vi "GetRefExample.vi"() -> ()   [LabVIEW 2019]
uses:
  _get control reference by name.vi
  _get mutiple control reference by name.vi
panel:
  in  "error in":errorcluster
  out "error out":errorcluster
  in  "Important Tab Control":enum32{"Page 1", "Page 2"}(tab)
  in  "Not So Important Path":path
  in  "Important String":string
  in  "Important Sub Tab Control":enum32{"Page 1", "Page 2"}(tab)
  out "Important Chart":dbl(graph)
  in  "Important Table":string[][](table)
  in  "Important Path":path
  in  "Important Button":bool
  in  "Important Number":dbl
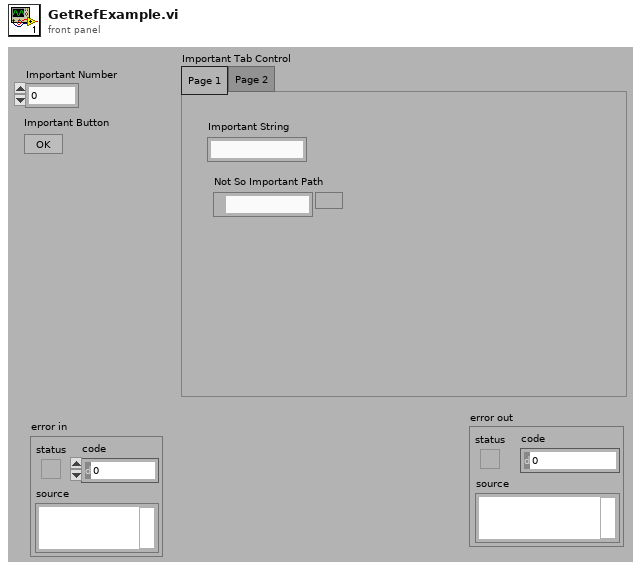
[diagram p1: front panel]
types:
  T1 = cluster{"ControlName":string, "ControlReference":refnum<vi>}[]
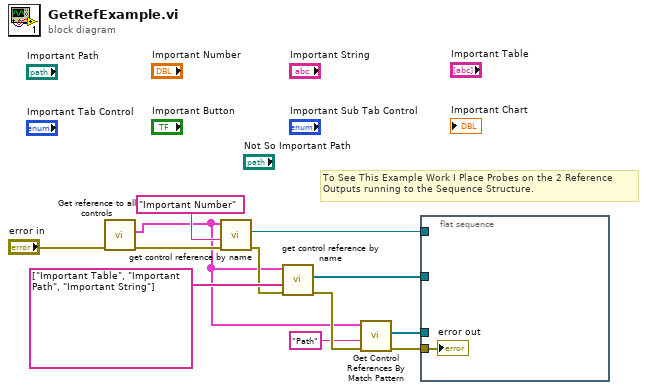
[diagram p0: block diagram]
diagram:
  # "To See This Example Work I Place Probes on the 2 Reference\nOutputs running to the Sequence Structure."
  n1 = call "Get reference to all controls.vi"("error in (no error)"="error in") -> ("error out"=w12:errorcluster, "Control references"=w2:T1)  [unwired: 5 in]
  n2 = call-poly "get control reference by name.vi"("error in (no error)"=w12, "Control name"="Important Number", "Control references"=w2) -> ("error out"=w8:errorcluster, "Ctl Refnum"=w10:refnum<vi>)  [unwired: 3 in]
  n3 = call-poly "get control reference by name.vi"("error in (no error)"=w8, "Control names"=string[] ["Important Table", "Important Path", "Important String"], "Control references"=w2) -> ("error out"=w5:errorcluster, "References"=w7:refnum<vi>[])  [unwired: 3 in]
  n4 = call "Get Control References By Match Pattern.vi"("error in (no error)"=w5, "regular expression"="Path", "Control references"=w2) -> ("error out"=w4:errorcluster, "References"=w3:refnum<vi>[])  [unwired: 3 in]
  n5 = flat-sequence {
    tunnel: w10 -> [_]
    tunnel: w7 -> [_]
    tunnel: w4 -> [w13]
    tunnel: w3 -> [_]
    frame #0 {
      "error out" <- w13
    }
  }
